vi "proceed.vi"(8 "error in (no error)":errorcluster, 11 "ScanModeMG090624Camera in":refnum<class "ImagingModeMG090624Camera.lvclass">) -> (0 "error out":errorcluster, 3 "ScanModeMG090624Camera out":refnum<class "ImagingModeMG090624Camera.lvclass">)   [LabVIEW 2010, in "ImagingModeMG090624Camera.lvclass"]
uses:
  ImagingModeMG090624Camera.lvclass
  ImagingModeMG090624Camera.lvclass/ImagingModeMG090624Camera.ctl
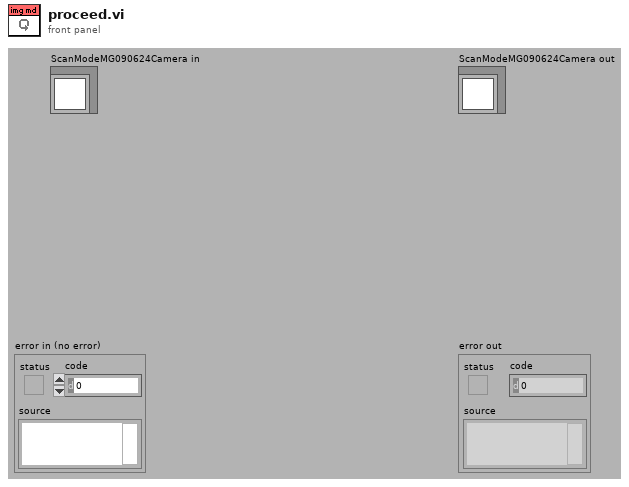
[diagram p1: front panel]
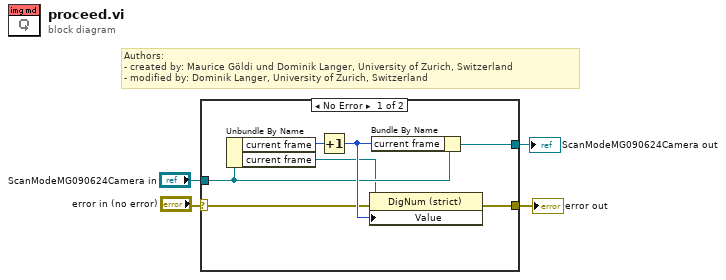
[diagram p0: block diagram]
diagram:
  # "Authors: \n- created by: Maurice Göldi und Dominik Langer, University of Zurich, Switzerland\n- modified by: Dominik Langer, University of Zurich, Switzerland"
  n1 = case shown="No Error" "error in (no error)" {
    selector: "error in (no error)" -> [w8 w13]
    tunnel: [w11 w13] -> w3
    tunnel: [w10 w12] -> w2
    tunnel: "ScanModeMG090624Camera in" -> [w7 w12]
    frame No Error {
      n2 = Unbundle By Name(w7) -> ("current frame"=w6:i32, "current frame"=w5:refnum<vi>)
      n3 = Increment(x=w6) -> (x+1=w9:i32)
      n4 = property class="DigNum (strict)"(reference=w5, error in=w8, "Value"=w9) -> (error out=w11:errorcluster)  [unwired: 1 out]
      n5 = Bundle By Name(cluster=w7, "current frame"=w9) -> (w10:refnum<class "ImagingModeMG090624Camera.lvclass">)
    }
    frame Error {
    }
  }
  "error out" <- w3
  "ScanModeMG090624Camera out" <- w2
